vi "Test Invalid Path Segment.vi"() -> ()   [LabVIEW 2020]
panel:
  out "error out":errorcluster
  out "String":string
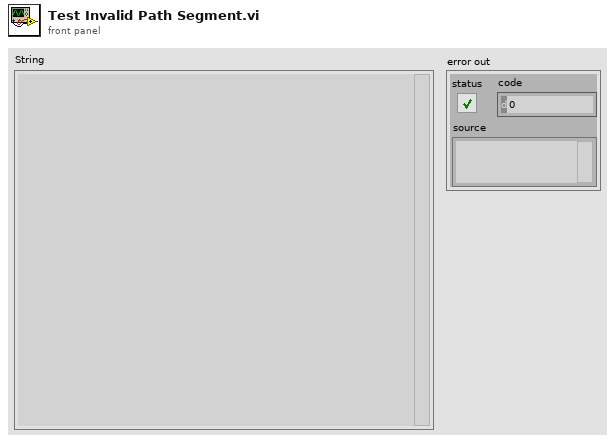
[diagram p1: front panel]
types:
  T1 = enum16{"Standard", "Buffered", "CRLF", "Immediate"}
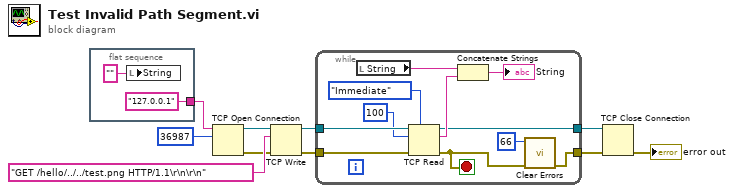
[diagram p0: block diagram]
diagram:
  n1 = flat-sequence {
    tunnel: ["127.0.0.1" ("address")] -> w10
    frame #0 {
      n2 = local write "String"("") -> ()
    }
  }
  n3 = TCP Open Connection(address=w10, remote port or service name=u16 36987) -> (connection ID=w8:refnum<k5>, error out=w6:errorcluster)  [unwired: 3 in]
  n4 = TCP Write(connection ID=w8, data in="GET /hello/../../test.png HTTP/1.1\r\n\r\n" ("url"), error in (no error)=w6) -> (connection ID out=w5:refnum<k5>, error out=w4:errorcluster)  [unwired: 1 in, 1 out]
  n5 = while {
    tunnel: w5 -> [w23]
    tunnel: w4 -> [w22]
    tunnel: [w13] -> w2
    tunnel: [w16] -> w3
    stop <- w15 stop-if-true
    n6 = local read "String"() -> (w19:string)
    n7 = TCP Read(connection ID=w23, bytes to read=100, error in (no error)=w22, 7:T1."Immediate" ("mode (standard)")) -> (connection ID out=w16:refnum<k5>, data out=w18:string, error out=w15:errorcluster)  [unwired: 1 in]
    n8 = Concatenate Strings(w19, w18) -> (→"String":string)
    n9 = call <vilib>:"Clear Errors.vi"("error in (no error)"=w15, "specific error code to clear (0: all)"=66) -> ("error out"=w13:errorcluster)  [unwired: 4 in, 1 out]
  }
  n10 = TCP Close Connection(connection ID=w3, error in (no error)=w2) -> (error out=→"error out":errorcluster)  [unwired: 1 in, 1 out]
